vi "UPS监控.vi"() -> ()   [LabVIEW 2016, in "环境动力监测库.lvlib" / "UPS库.lvlib"]
uses:
  <vilib>/Utility/miscctls.llb/LVPointTypeDef.ctl
panel:
  in  "变更UPS型号":bool
  out "布尔":bool
  # "UPS监测"
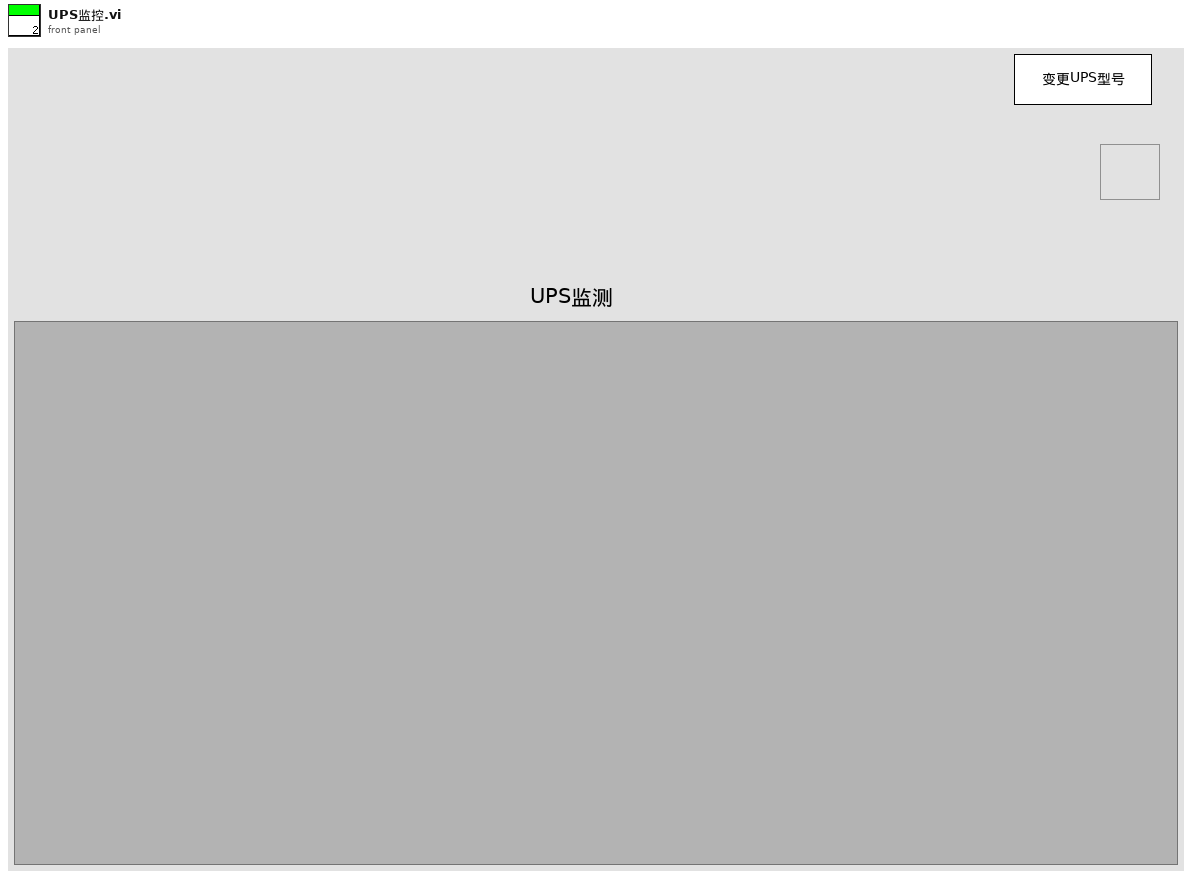
[diagram p1: front panel]
types:
  T1 = enum16{"报警状态监测", "报警确认", "仪器断电", "工控机关机", "取消告警", "结束"}
  T2 = typedef "LVPointTypeDef.ctl" = cluster{"Horizontal":i16, "Vertical":i16}
  T3 = typedef "环境动力监测库.lvlib/UPS库.lvlib/UPS型号.ctl" = enum16{"山特UPSC1~3", "山特UPSC6~20", "华为UPS2000-G-(1-3KVA)", "Kstar"}
  T4 = cluster{"VISA resource name":refnum<visa-resource-name>, "Serial Config":cluster{"baud rate (9600)":u32, "stop bits (10: 1 bit)":u16, "parity (0:none)":enum16{"None", "Odd", "Even", "Mark", "Space"}, "data bits (8)":u16, "timeout (10sec)":u32}, "型号选择":T3, "HW-UPS-2000 MB session":refnum<class "MB_Master.lvclass">, "连接方式":enum16{"串口", "TCP"}, "IP":string, "Port":string, "低电量报警阈值":u16, "功能启用":bool}
  T5 = enum32{"Bad", "Idle", "Run top level", "Running"}
  T6 = cluster{"输入电压R":dbl, "输入电压S":dbl, "输入电压T":dbl, "输入频率":dbl, "输出电压R":dbl, "输出电压S":dbl, "输出电压T":dbl, "输出频率":dbl, "输出电流R":dbl, "输出电流S":dbl, "输出电流T":dbl, "Positive电池电压":dbl, "Negative电池电压":dbl, "温度":dbl, "电池剩余备用时间":dbl, "电池容量百分比":dbl, "系统模式":dbl, "电池测试状态":dbl, "故障代码":string, "告警":string}
  T7 = cluster{"电池电压V":dbl, "电池状态":u16, "电池剩余容量%":u16, "电池后备时间s":u32, "电池节数":u16, "电池容量AH":u16, "UPS机型KVA":u16}
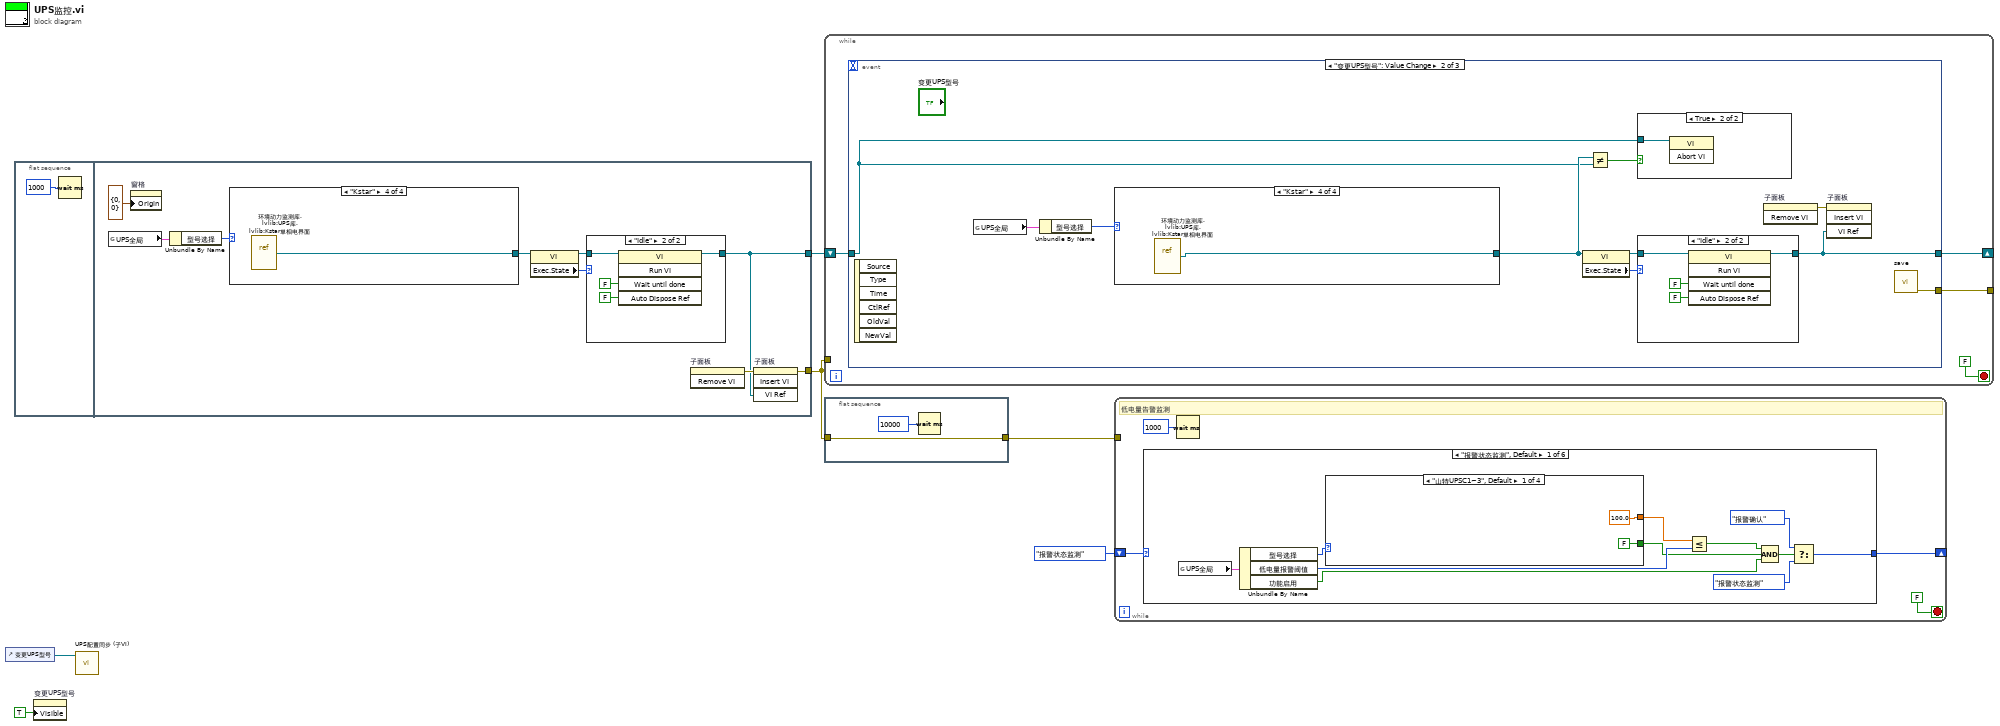
[diagram p0: block diagram]
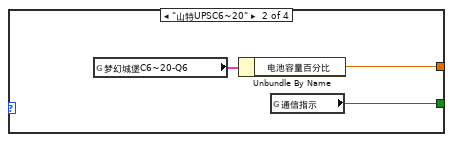
[diagram p2: hidden frame]
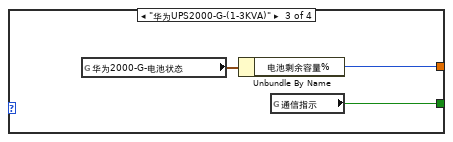
[diagram p3: hidden frame]
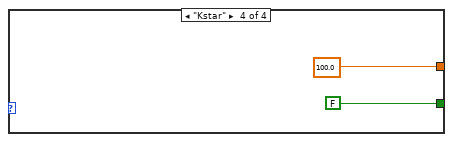
[diagram p4: hidden frame]
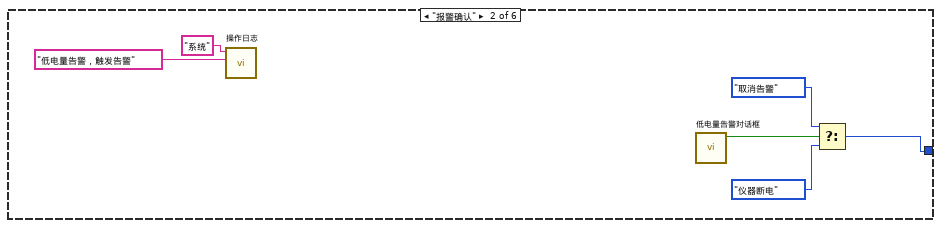
[diagram p5: hidden frame]
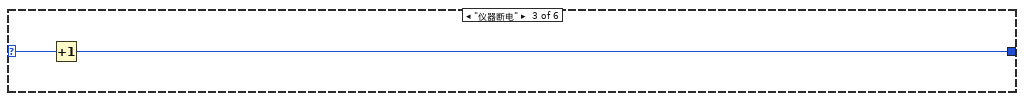
[diagram p6: hidden frame]
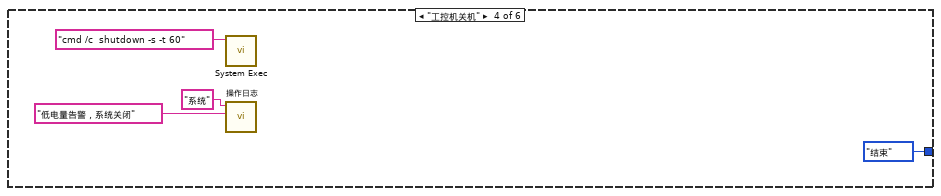
[diagram p7: hidden frame]
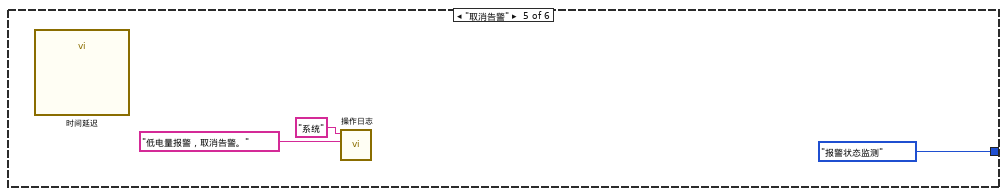
[diagram p8: hidden frame]
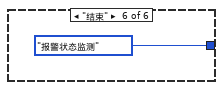
[diagram p9: hidden frame]
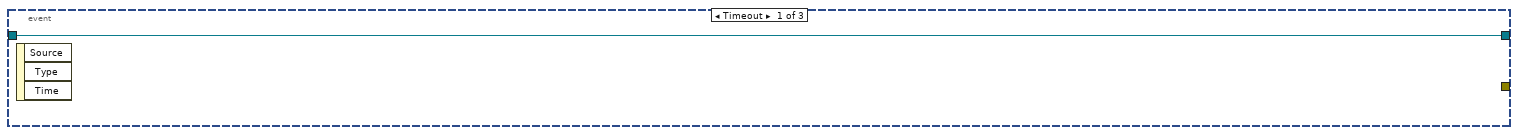
[diagram p10: hidden frame]
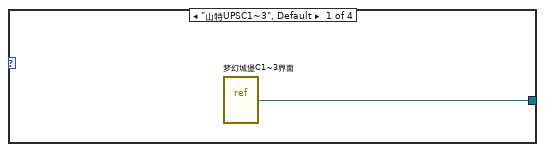
[diagram p12: hidden frame]
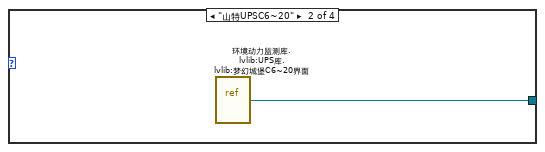
[diagram p13: hidden frame]
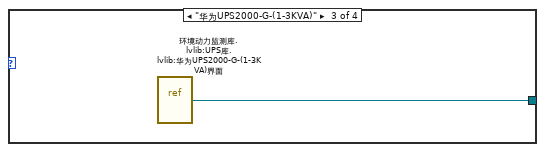
[diagram p14: hidden frame]
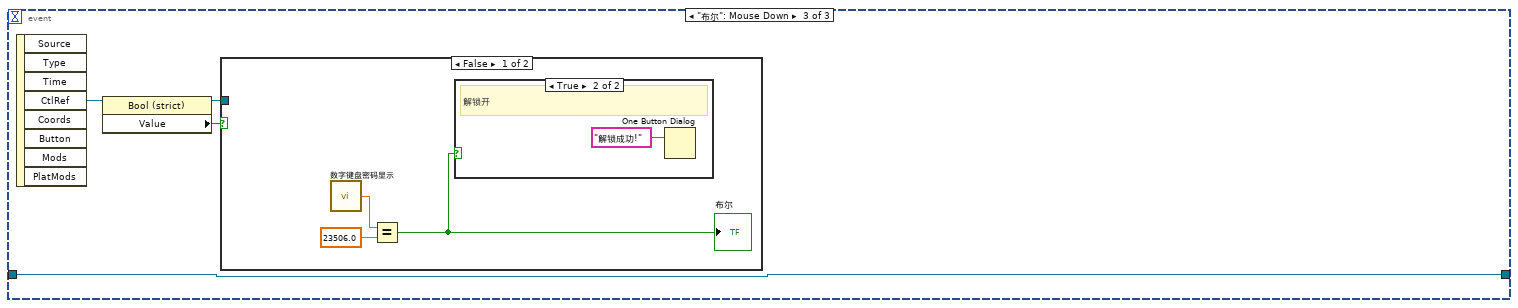
[diagram p16: hidden frame]
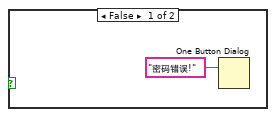
[diagram p17: hidden frame]
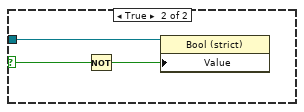
[diagram p18: hidden frame]
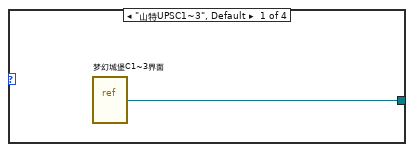
[diagram p19: hidden frame]
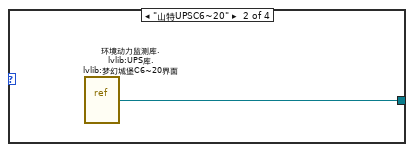
[diagram p20: hidden frame]
diagram:
  n1 = control-ref of="变更UPS型号"() -> (w5:refnum<vi>)
  n2 = flat-sequence {
    tunnel: [w12] -> w2
    tunnel: [w11] -> w6
    frame #0 {
      n3 = Wait (ms)(milliseconds to wait=u32 1000 ("等待时间（毫秒）")) -> ()  [unwired: 1 out]
    }
    frame #1 {
      n4 = global read "断电保存全局变量.vi" "UPS全局"() -> (w9:T4)
      n5 = property on="窗格" class="Pane"("Origin"=T2 {"Horizontal"=0, "Vertical"=0} ("原点")) -> ()  [unwired: 2 in, 2 out]
      n6 = Unbundle By Name(w9) -> ("型号选择"=w8:T3)
      n7 = case shown="\"Kstar\"" w8 {
        tunnel: [w17 w18 w19 w20] -> w14
        frame "山特UPSC1~3", Default {
          n8 = vi-ref "梦幻城堡C1~3界面.vi"() -> (w17:refnum<vi>)
        }
        frame "山特UPSC6~20" {
          n9 = vi-ref "环境动力监测库.lvlib:UPS库.lvlib:梦幻城堡C6~20界面.vi"() -> (w18:refnum<vi>)
        }
        frame "华为UPS2000-G-(1-3KVA)" {
          n10 = vi-ref "环境动力监测库.lvlib:UPS库.lvlib:华为UPS2000-G-(1-3KVA)界面.vi"() -> (w19:refnum<vi>)
        }
        frame "Kstar" {
          n11 = vi-ref "环境动力监测库.lvlib:UPS库.lvlib:Kstar单相电界面.vi"() -> (w20:refnum<vi>)
        }
      }
      n12 = property class="VI"(reference=w14) -> (reference out=w15:refnum<vi>, "Exec.State"=w16:T5)  [unwired: 1 in, 1 out]
      n13 = case shown="\"Idle\"" w16 {
        tunnel: w15 -> [w21 w23]
        tunnel: [w21 w22] -> w11
        frame "Bad", Default {
        }
        frame "Idle" {
          n14 = invoke class="VI" method="Run VI"(reference=w23, "Wait until done"=FALSE ("结束前等待"), "Auto Dispose Ref"=FALSE ("自动销毁引用")) -> (reference out=w22:refnum<vi>)  [unwired: 2 in, 4 out]
        }
      }
      n15 = invoke on="子面板" class="SubPnl" method="Remove VI"() -> (error out=w13:errorcluster)  [unwired: 3 in, 2 out]
      n16 = invoke on="子面板" class="SubPnl" method="Insert VI"(error in=w13, "VI Ref"=w11) -> (error out=w12:errorcluster)  [unwired: 2 in, 3 out]
    }
  }
  n17 = property on="变更UPS型号" class="Bool (严格)"("Visible"=TRUE ("可见")) -> ()  [unwired: 2 in, 2 out]
  n18 = call "UPS配置同步 (子VI).vi"("Boolean输入"=w5) -> ()  [unwired: 11 in]
  n19 = while {
    tunnel: w2 -> [_]
    tunnel: [w29] -> _
    shift-right: [w26] -> _
    shift-left: w6 -> [w28]
    stop <- FALSE stop-if-true
    n20 = event shown="[1] \"变更UPS型号\": Value Change" {
      selector: _ -> [_ _ _]
      dyn-events: _ -> [_ _ _]
      timeout: _ -> [_ _ _]
      tunnel: [_ w33 _] -> w29
      tunnel: w28 -> [w30 w34 w51]
      tunnel: [w30 w40 w51] -> w26
      event Timeout {
        n21 = event-data() -> ()  [unwired: 1 in, 3 out]
      }
      event "变更UPS型号": Value Change {
        n22 = event-data() -> ()  [unwired: 1 in, 6 out]
        n23 = global read "断电保存全局变量.vi" "UPS全局"() -> (w32:T4)
        n24 = Unbundle By Name(w32) -> ("型号选择"=w31:T3)
        n25 = case shown="\"Kstar\"" w31 {
          tunnel: [w42 w43 w44 w45] -> w36
          frame "山特UPSC1~3", Default {
            n26 = vi-ref "梦幻城堡C1~3界面.vi"() -> (w42:refnum<vi>)
          }
          frame "山特UPSC6~20" {
            n27 = vi-ref "环境动力监测库.lvlib:UPS库.lvlib:梦幻城堡C6~20界面.vi"() -> (w43:refnum<vi>)
          }
          frame "华为UPS2000-G-(1-3KVA)" {
            n28 = vi-ref "环境动力监测库.lvlib:UPS库.lvlib:华为UPS2000-G-(1-3KVA)界面.vi"() -> (w44:refnum<vi>)
          }
          frame "Kstar" {
            n29 = vi-ref "环境动力监测库.lvlib:UPS库.lvlib:Kstar单相电界面.vi"() -> (w45:refnum<vi>)
          }
        }
        n30 = property class="VI"(reference=w36) -> (reference out=w38:refnum<vi>, "Exec.State"=w39:T5)  [unwired: 1 in, 1 out]
        n31 = Not Equal?(x=w36, y=w34) -> (x != y?=w35:bool)
        n32 = case shown="True" w35 {
          tunnel: w34 -> [_ w41]
          frame False {
          }
          frame True {
            n33 = invoke class="VI" method="Abort VI"(reference=w41) -> ()  [unwired: 2 in, 3 out]
          }
        }
        n34 = case shown="\"Idle\"" w39 {
          tunnel: w38 -> [w46 w48]
          tunnel: [w46 w47] -> w40
          frame "Bad", Default {
          }
          frame "Idle" {
            n35 = invoke class="VI" method="Run VI"(reference=w48, "Wait until done"=FALSE ("结束前等待"), "Auto Dispose Ref"=FALSE ("自动销毁引用")) -> (reference out=w47:refnum<vi>)  [unwired: 2 in, 4 out]
          }
        }
        n36 = invoke on="子面板" class="SubPnl" method="Remove VI"() -> (error out=w37:errorcluster)  [unwired: 3 in, 2 out]
        n37 = invoke on="子面板" class="SubPnl" method="Insert VI"(error in=w37, "VI Ref"=w40) -> ()  [unwired: 2 in, 4 out]
        n38 = call "save.vi"() -> ("error out"=w33:errorcluster)  [unwired: 11 in]
      }
      event "布尔": Mouse Down {
        n39 = event-data() -> ("CtlRef"=w54:refnum<vi>)  [unwired: 1 in, 7 out]
        n40 = property class="Bool (strict)"(reference=w54) -> (reference out=w52:refnum<vi>, "Value"=w53:bool)  [unwired: 1 in, 1 out]
        n41 = case shown="False" w53 {
          selector: w53 -> [_ w61]
          tunnel: w52 -> [_ w62]
          frame False {
            n42 = call "数字键盘密码显示.vi"() -> ("NewNumber"=w57:sgl)  [unwired: 1 in]
            n43 = Equal?(x=w57, y=sgl 23506.0) -> (x = y?=w55:bool)
            "布尔" <- w55
            n44 = case shown="True" w55 {
              frame False {
                n45 = One Button Dialog(message="密码错误!" ("消息")) -> ()  [unwired: 1 in, 1 out]
              }
              frame True {
                # "解锁开"
                n46 = One Button Dialog(message="解锁成功!" ("消息")) -> ()  [unwired: 1 in, 1 out]
              }
            }
          }
          frame True {
            n47 = Not(x=w61) -> (.not. x?=w60:bool)
            n48 = property class="Bool (strict)"(reference=w62, "Value"=w60) -> ()  [unwired: 1 in, 2 out]
          }
        }
      }
    }
  }
  n49 = flat-sequence {
    tunnel: w2 -> [w64]
    tunnel: [w64] -> w1
    frame #0 {
      n50 = Wait (ms)(milliseconds to wait=u32 10000 ("等待时间（毫秒）")) -> ()  [unwired: 1 out]
    }
  }
  n51 = while {
    shift-right: [w68] -> _
    shift-left: T1."报警状态监测" ("枚举") -> [w67]
    tunnel: w1 -> [_]
    stop <- FALSE stop-if-true
    # "低电量告警监测"
    n52 = case shown="\"报警状态监测\", Default" w67 {
      selector: w67 -> [_ _ w97 _ _ _]
      tunnel: [w72 w92 w96 T1."结束" ("枚举") T1."报警状态监测" ("枚举") T1."报警状态监测" ("枚举")] -> w68
      frame "报警状态监测", Default {
        n53 = global read "断电保存全局变量.vi" "UPS全局"() -> (w79:T4)
        n54 = Unbundle By Name(w79) -> ("型号选择"=w78:T3, "低电量报警阈值"=w76:u16, "功能启用"=w69:bool)
        n55 = case shown="\"山特UPSC1~3\", Default" w78 {
          tunnel: [100.0 ("电池容量百分比") w83 w86 100.0 ("电池容量百分比")] -> w77
          tunnel: [FALSE ("通信指示") w82 w85 FALSE ("通信指示")] -> w70
          frame "山特UPSC1~3", Default {
          }
          frame "山特UPSC6~20" {
            n56 = global read "UPS内部交互全局.vi" "梦幻城堡C6~20-Q6"() -> (w84:T6)
            n57 = Unbundle By Name(w84) -> ("电池容量百分比"=w83:dbl)
            n58 = global read "UPS内部交互全局.vi" "通信指示"() -> (w82:bool)
          }
          frame "华为UPS2000-G-(1-3KVA)" {
            n59 = global read "UPS内部交互全局.vi" "华为2000-G-电池状态"() -> (w87:T7)
            n60 = Unbundle By Name(w87) -> ("电池剩余容量%"=w86:u16)
            n61 = global read "UPS内部交互全局.vi" "通信指示"() -> (w85:bool)
          }
          frame "Kstar" {
          }
        }
        n62 = Less Or Equal?(x=w77, y=w76) -> (x <= y?=w75:bool)
        n63 = Compound Arithmetic op=AND ("复合运算")(w75, w70, w69) -> (w71:bool)
        n64 = Select(t=T1."报警确认" ("枚举"), s=w71, f=T1."报警状态监测" ("枚举")) -> (s? t:f=w72:T1)
      }
      frame "报警确认" {
        n65 = call "操作日志.vi"("日志信息"="低电量告警，触发告警", "设备"="系统") -> ()  [unwired: 9 in, 1 out]
        n66 = call "低电量告警对话框.vi"() -> ("T button?"=w95:bool)  [unwired: 11 in]
        n67 = Select(t=T1."取消告警" ("枚举"), s=w95, f=T1."仪器断电" ("枚举")) -> (s? t:f=w92:T1)
      }
      frame "仪器断电" {
        n68 = Increment(x=w97) -> (x+1=w96:T1)
      }
      frame "工控机关机" {
        n69 = call <vilib>:"System Exec.vi"("command line"="cmd /c  shutdown -s -t 60") -> ()  [unwired: 7 in, 4 out]
        n70 = call "操作日志.vi"("日志信息"="低电量告警，系统关闭", "设备"="系统") -> ()  [unwired: 9 in, 1 out]
      }
      frame "取消告警" {
        n71 = call "时间延迟"() -> ()  [unwired: 11 in, 1 out]
        n72 = call "操作日志.vi"("日志信息"="低电量报警，取消告警。", "设备"="系统") -> ()  [unwired: 9 in, 1 out]
      }
      frame "结束" {
      }
    }
    n73 = Wait (ms)(milliseconds to wait=u32 1000 ("等待时间（毫秒）")) -> ()  [unwired: 1 out]
  }
